vi "Set main VI busy cursor.vi"(8 "error in (no error)":errorcluster, 11 "Main VI's cursor":T1) -> (0 "error out":errorcluster)   [LabVIEW 2013]
uses:
  Typedefs/Set Main VI cursor.ctl
  Global Variables/gl_UI Ctrl Refs.vi
panel:
  out "call chain release":string[](array[string])
  out "call chain set":string[](array[string])
  out "Release":u32
  out "Set":u32
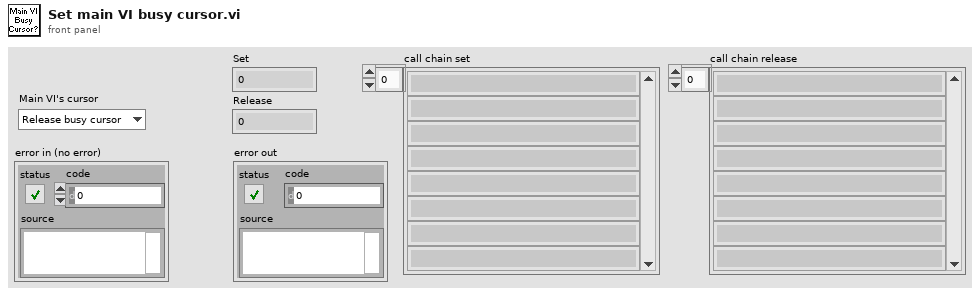
[diagram p1: front panel]
types:
  T1 = typedef "Set Main VI cursor.ctl" = enum16{"Release busy cursor", "Set busy cursor"}
  T2 = typedef "UI ctrl refs cluster.ctl" = cluster{"Top level VI path":path, "Top level VI ref":refnum<vi>, "User menu ref":refnum<k9>, "Sub Panel control":refnum<vi>, "Imaging Param Tab":refnum<vi>, "Occurrence-Start drivers":refnum<k4>, "Occurrence-Speed logging initialised":refnum<k4>, "Occurrence-XYZ stage initialised":refnum<k4>, "Exit button":refnum<vi>, "Status ind":refnum<vi>, "Return to Origin":refnum<vi>, "Speed Logging":refnum<vi>, "Time Lapse":refnum<vi>, "Live Imaging":refnum<vi>, "AOL Z Stack":refnum<vi>, "Motor Z Stack":refnum<vi>, "Funct Acq button":refnum<vi>, "Hard Shutter":refnum<vi>, "Virtual Shutter":refnum<vi>, "Laser Power":refnum<vi>, "AOL Mode":refnum<vi>, "Frame Size":refnum<vi>, "Field of View":refnum<vi>, "Dwell Time":refnum<vi>, "Zoom":refnum<vi>, "AOL Z":refnum<vi>, "Objective":refnum<vi>, "Axis":refnum<vi>, "Paths & Names":refnum<vi>, "Experiment folder path (ind.)":refnum<vi>, "Last State (Ind.)":refnum<vi>, "Laser wavelength ind (nm)":refnum<vi>, "Averages":refnum<vi>, "Angle (degrees)":refnum<vi>, "X centre":refnum<vi>, "Y centre":refnum<vi>, "Plane Mode":refnum<vi>, "# Planes":refnum<vi>, "Z Start":refnum<vi>, "Z Stop":refnum<vi>, "Z Step":refnum<vi>, "PMT 1":refnum<vi>, "PMT 2":refnum<vi>, "Stage XYZ Position":refnum<vi>, "Pockels@Z Start":refnum<vi>, "Pockels@Z Stop":refnum<vi>, "Obtain Z Start":refnum<vi>, "Obtain Z Stop":refnum<vi>, "Live stim.trig.period":refnum<vi>, "Live stim.trig.enable":refnum<vi>, "Funct. Acq. Pockels Modulation":refnum<vi>, "Enable Video Recording":refnum<vi>, "Video Record-Live Imaging":refnum<vi>, "Video Record-Funct acq":refnum<vi>, "AOL Z-stack Chirps Ready (ind)":refnum<vi>, "Center freq ind (nm)":refnum<vi>, "Logging queue (ind)":refnum<vi>, "Back aperture power (ind.)":refnum<vi>, "Power after objective (ind.)":refnum<vi>, "Switch user":refnum<vi>}
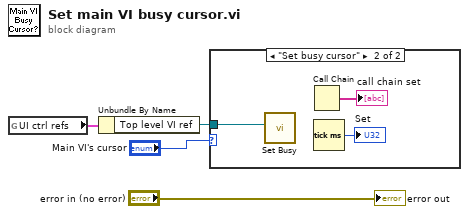
[diagram p0: block diagram]
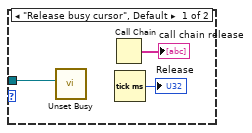
[diagram p2: hidden frame]
diagram:
  n1 = global read "gl_UI Ctrl Refs.vi" "UI ctrl refs"() -> (w2:T2)
  n2 = Unbundle By Name(w2) -> ("Top level VI ref"=w3:refnum<vi>)
  n3 = case shown="\"Set busy cursor\"" "Main VI's cursor" {
    tunnel: w3 -> [w7 w10]
    frame "Release busy cursor", Default {
      n4 = call <vilib>:"Unset Busy.vi"("VI reference (current VI)"=w7) -> ()  [unwired: 10 in, 1 out]
      n5 = Call Chain() -> (call chain=→"call chain release":string[])
      n6 = Tick Count (ms)() -> (millisecond timer value=→"Release":u32)
    }
    frame "Set busy cursor" {
      n7 = call <vilib>:"Set Busy.vi"("VI reference (current VI)"=w10) -> ()  [unwired: 9 in, 2 out]
      n8 = Call Chain() -> (call chain=→"call chain set":string[])
      n9 = Tick Count (ms)() -> (millisecond timer value=→"Set":u32)
    }
  }
  "error out" <- "error in (no error)"
